vi "Calc Inputs.vi"(8 "error in (no error)":errorcluster, 11 "Median Calc in":refnum<class "Median Calc.lvclass">) -> (0 "error out":errorcluster, 2 "Inputs":string[](array[string]))   [LabVIEW 2020, in "VolatusCalcs.lvlib" / "Median Calc.lvclass"]
uses:
  Median Calc.lvclass
  Median Calc.lvclass/Median Calc.ctl
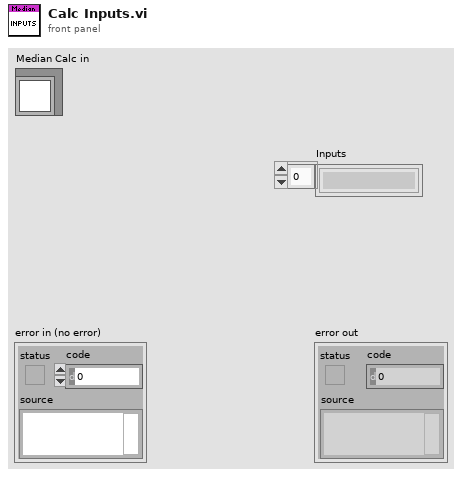
[diagram p1: front panel]
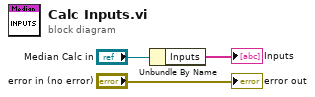
[diagram p0: block diagram]
diagram:
  n1 = Unbundle By Name("Median Calc in") -> ("Inputs"=→"Inputs":string[])
  "error out" <- "error in (no error)"
